vi "PH_ImageOperator.PC Set Energy Settings.vi"(0 "i ref in":refnum<vi>, 2 "Calc Energy":bool, 3 "Expected Value [mJ]":dbl, 4 "Tolerance [%]":dbl, 5 "error in (no error)":errorcluster) -> (14 "i ref out":refnum<vi>, 19 "error out":errorcluster)   [LabVIEW 2014, in "PH_ImageOperator.lvlib"]
doc: "This VI writes the energy settings to own attributes and sets the GUI elements."
uses:
  PH_ImageOperator.lvlib
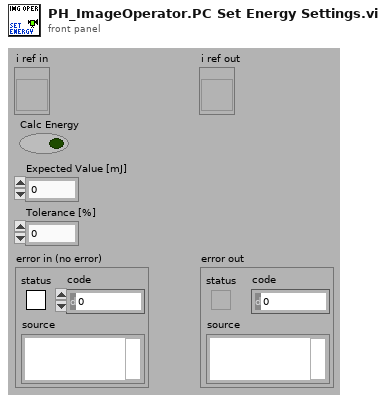
[diagram p1: front panel]
types:
  T1 = typedef "PH_ImageOperator.lvlib/PH_ImageOperator.i attribute.ctl" = cluster{"GUI Refs":cluster{"Delete":refnum<vi>, "Calibration status":refnum<vi>, "BI subtracted":refnum<vi>, "calc Energy":refnum<vi>, "Energy: expected value":refnum<vi>, "Energy: Tolerance":refnum<vi>, "Energy calculated":refnum<vi>, "Energy":refnum<vi>, "calc Beam Anal":refnum<vi>, "Maj Diam 1/esquare":refnum<vi>, "Min Diam 1/esquare":refnum<vi>, "Azi Angle":refnum<vi>, "Min/Maj Diam esquare":refnum<vi>, "Beam analysed":refnum<vi>, "CoG - x":refnum<vi>, "CoG - y":refnum<vi>, "BA: Method":refnum<vi>, "BA: Steps":refnum<vi>, "BA: Factor":refnum<vi>, "calc Traces":refnum<vi>, "Traces: Fit Gauss":refnum<vi>, "Traces calculated":refnum<vi>, "Maj FWHM":refnum<vi>, "Min FWHM":refnum<vi>, "Major Trace":refnum<vi>, "Minor Trace":refnum<vi>, "Maj Fit Order":refnum<vi>, "Min Fit Order":refnum<vi>, "Position calculated":refnum<vi>, "Position":refnum<vi>, "Type":refnum<vi>, "Center":refnum<vi>, "exp - X":refnum<vi>, "exp - Y":refnum<vi>, "Tolerance":refnum<vi>, "f":refnum<vi>, "M":refnum<vi>, "D":refnum<vi>, "q":refnum<vi>, "Dummy Method":refnum<vi>, "Dummy Type":refnum<vi>, "Global On":refnum<vi>, "Traces: No offset":refnum<vi>, "Maj 99%":refnum<vi>, "Min 99%":refnum<vi>, "GUI FF Image":refnum<vi>, "calc Fill Factor":refnum<vi>, "FF calculated":refnum<vi>, "Fill Factor: Filter?":refnum<vi>, "FF: Damage Threshold":refnum<vi>, "FF: Threshold":refnum<vi>, "FF: max allow. Energy":refnum<vi>, "FF: Fillfactor":refnum<vi>, "Calibration data":refnum<vi>}, "List of GUIs":string[], "Calibration":cluster{"Status":T2, "Calibration data":T3, "Calibration Data File":path}, "Final Image":cluster{"BI Subtraction Failure":bool}, "Energy":cluster{"on":bool, "expected value [mJ]":dbl, "Tolerance [%]":dbl, "State":T2, "Energy [mJ]":dbl, "Unit":string, "calculated @":timestamp}, "Beam Analysis":cluster{"on":bool, "Data":T4, "Method":bool, "Steps":i32, "Factor":i32, "ROI":cluster{"Left":i32, "Top":i32, "Right":i32, "Bottom":i32}, "analysed @":timestamp}, "Trace Analysis":cluster{"on":bool, "Fit on":bool, "Maj FWHM":dbl, "Min FWHM":dbl, "Maj Fit Order":i32, "Min Fit Order":i32, "No Offset":bool, "Maj 99%":dbl, "Min 99%":dbl, "Traces":cluster{"XScaleName":string, "Y Scale Minimum":sgl, "Y Scale Maximum":sgl, "X Scale Minimum":sgl, "X Scale Maximum":sgl, "Traces":cluster{"Index":sgl[], "Trace":dbl[]}[]}[], "analysed @":timestamp}, "Position Analysis":cluster{"on":bool, "exp - X":i32, "exp - Y":i32, "focal length [mm]":dbl, "Magnification":dbl, "Delta":dbl, "Theta":dbl, "Tolerance":dbl, "Type":bool, "analysed @":timestamp}, "Fill Factor":cluster{"on":bool, "Filter on?":bool, "Threshold":dbl, "Damage Threshold [J/cm²]":dbl, "Fillfactor":dbl, "Max. allowed Energy [J]":dbl, "calculated @":timestamp}, "Statistician Service ID":i32, "Images":cluster{"Background":T5, "OP":T5, "GUI":T5, "BA: ROI":T5, "Trace: Turn":T5, "FF: Main":T5, "FF: Help":T5, "PSDB: BG":T5, "PSDB: OP":T5, "PSDB: FF":T5}}
  T2 = typedef "PH_StatusHandler.lvlib/PH_StatusHandler.Status.ctl" = i16
  T3 = typedef "PH_ImageCalibrator.lvlib/PH_ImageCalibrator.Calibration Data.ctl" = cluster{"Date":string, "Time":string, "Cam Settings":cluster{"Cam ID":string, "Gain":dbl, "Brightness":dbl, "Shutter":dbl, "Cam Error":bool, "Mode":i32}, "Background Image":cluster{"Image":dbl[][], "Image Error":bool}, "Linear Calibration":cluster{"Calibration Factor":dbl, "not mm or mrad":bool}, "Energy Calibration":cluster{"Calibration Factor":dbl, "no mJ":bool}}
  T4 = typedef "PH_ImageOperator.lvlib/PH_ImageOperator.Beam Analysis Data.ctl" = cluster{"CoG-x":sgl, "CoG-y":sgl, "Maj Dim":dbl, "Min Dim":dbl, "Ellipticity":dbl, "Azimuth Angle [rad]":dbl, "Azi Angle rel to Maj?":bool}
  T5 = typedef "IMAQ Image.ctl" = refnum<image>
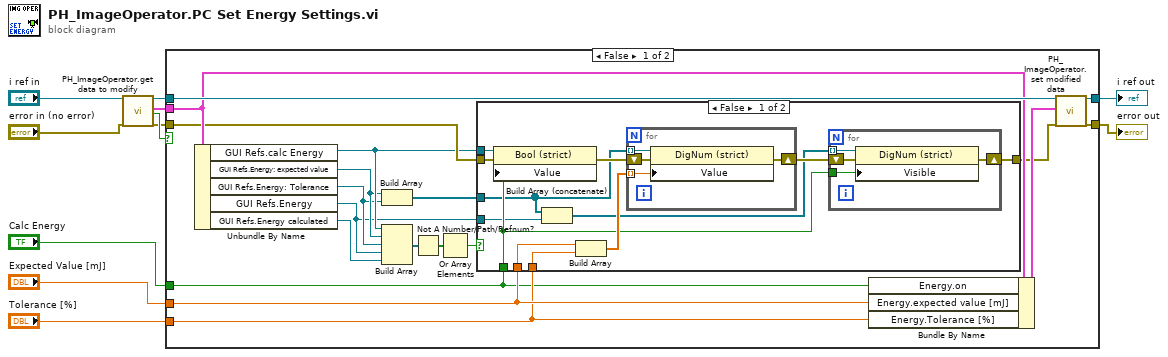
[diagram p0: block diagram]
diagram:
  n1 = call "PH_ImageOperator.get data to modify.vi"("i ref in"="i ref in", "error in (no error)"="error in (no error)") -> ("i ref out"=w3:refnum<vi>, "i attribute"=w8:T1, "timed out"=w7:bool, "error out"=w2:errorcluster)  [unwired: 14 in]
  n2 = case shown="False" w7 {
    tunnel: w2 -> [w25 w52]
    tunnel: w3 -> [w30 w53]
    tunnel: [w29 w53] -> w4
    tunnel: [w28 w52] -> w6
    tunnel: w8 -> [w26 _]
    tunnel: "Calc Energy" -> [w14 _]
    tunnel: "Expected Value [mJ]" -> [w16 _]
    tunnel: "Tolerance [%]" -> [w15 _]
    frame False {
      n3 = Unbundle By Name(w26) -> ("GUI Refs.calc Energy"=w23:refnum<vi>, "GUI Refs.Energy: expected value"=w19:refnum<vi>, "GUI Refs.Energy: Tolerance"=w18:refnum<vi>, "GUI Refs.Energy"=w13:refnum<vi>, "GUI Refs.Energy calculated"=w12:refnum<vi>)
      n4 = Build Array(w19, w18) -> (w17:refnum<vi>[])
      n5 = Build Array(w23, w19, w18, w13, w12) -> (w22:refnum<vi>[])
      n6 = Not A Number/Path/Refnum?(number/path/refnum=w22) -> (NaN/Path/Refnum?=w21:bool[])
      n7 = Or Array Elements(Boolean array=w21) -> (logical OR=w20:bool)
      n8 = case shown="False" w20 {
        tunnel: w25 -> [w42 w51]
        tunnel: [w34 w51] -> w24
        tunnel: w23 -> [w41 _]
        tunnel: w14 -> [w35 _]
        tunnel: w17 -> [w32 _]
        tunnel: w16 -> [w39 _]
        tunnel: w15 -> [w38 _]
        tunnel: w13 -> [w33 _]
        frame False {
          n9 = property class="Bool (strict)"(reference=w41, error in=w42, "Value"=w35) -> (error out=w40:errorcluster)  [unwired: 1 out]
          n10 = Build Array (concatenate)(w32, w33) -> (w31:refnum<vi>[])
          n11 = Build Array(w39, w38) -> (w37:dbl[])
          n12 = for {
            shift-right: [w49] -> w36
            shift-left: w40 -> [w50]
            tunnel: w32 -> [w48] mode=indexing
            tunnel: w37 -> [w47] mode=indexing
            n13 = property class="DigNum (strict)"(reference=w48, error in=w50, "Value"=w47) -> (error out=w49:errorcluster)  [unwired: 1 out]
          }
          n14 = for {
            tunnel: w35 -> [w45]
            tunnel: w31 -> [w43] mode=indexing
            shift-right: [w44] -> w34
            shift-left: w36 -> [w46]
            n15 = property class="DigNum (strict)"(reference=w43, error in=w46, "Visible"=w45) -> (error out=w44:errorcluster)  [unwired: 1 out]
          }
        }
        frame True {
        }
      }
      n16 = Bundle By Name(cluster=w26, "Energy.on"=w14, "Energy.expected value [mJ]"=w16, "Energy.Tolerance [%]"=w15) -> (w27:T1)
      n17 = call "PH_ImageOperator.set modified data.vi"("i ref in"=w30, "i attribute"=w27, "error in (no error)"=w24) -> ("i ref out"=w29:refnum<vi>, "error out"=w28:errorcluster)  [unwired: 15 in]
    }
    frame True {
    }
  }
  "error out" <- w6
  "i ref out" <- w4
